vi "Read (Single Waveform).vi"(0 "VISA resource name":refnum<visa-resource-name>, 1 "Segment Index (0)":i32 format="%.0g", 5 "Measurement Source (1: Channel 1)":i32(ring)=1 items=["Channel 1"=1, "Channel 2"=2, "Channel 3"=3, "Channel 4"=4, "Function 1"=5, "Function 2"=6, "Function 3"=7, "Function 4"=8, "Memory 1"=9, "Memory 2"=10, "Memory 3"=11, "Memory 4"=12], 9 "Maximum Time (100000ms)":u32=100000, 11 "error in (no error)":errorcluster) -> (4 "VISA resource name out":refnum<visa-resource-name>, 8 "Waveform Data":waveform(dbl)(graph), 15 "error out":errorcluster)   [LabVIEW 2020, in "Agilent 90000 Series.lvlib"]
doc: "Initiates an acquisition on all channels that you enabled with the Configure Channel VI. The VI waits for the acquisition to complete and returns the waveform for the <B>Measurement Source</B> you specified. If the oscilloscope did not complete the acquisition within the time period you specify with the <B>Maximum Time</B> control, the VI returns a timeout error. A common cause for a timeout error is the acquisition was not triggered. For example, the trigger level is out of range of the waveform. If the sampling mode is set to segment, you can set the <B>Segment Index</B>.\n\nCall the Fetch (Single Waveform) VI to obtain the waveforms for each of the remaining enabled channels without initiating another acquisition.\n\n<B>Note:</B> If your instrument does not support auto compensation for probe attenuation, you may need to adjust the scaling of the Waveform Data accordingly. This is handled automatically in the <B>Configure Channel</B> VI or can be done manually by multiplying the <B>Waveform Data</B> by the probe attenuation."
uses:
  Agilent 90000 Series.lvlib
  Low Level/Fetch (Waveform).vi
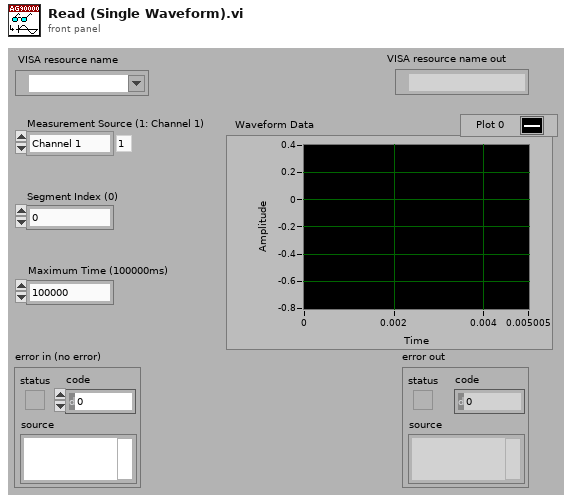
[diagram p1: front panel]
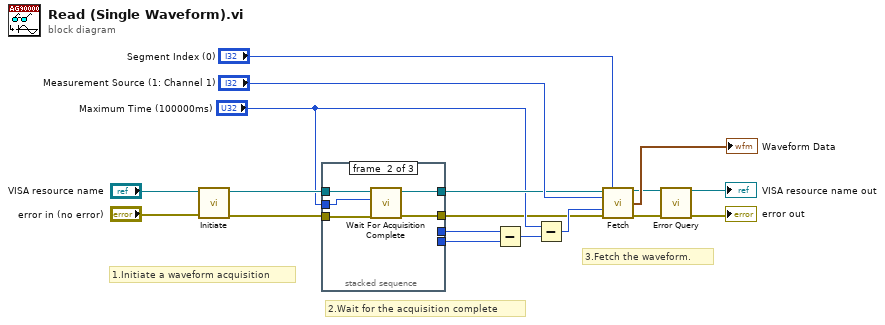
[diagram p0: block diagram]
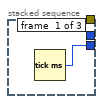
[diagram p2: hidden frame]
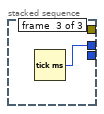
[diagram p3: hidden frame]
diagram:
  # "3.Fetch the waveform."
  # "2.Wait for the acquisition complete"
  # "1.Initiate a waveform acquisition"
  n1 = call "Initiate.vi"("error in (no error)"="error in (no error)", "VISA resource name"="VISA resource name") -> ("error out"=w8:errorcluster, "VISA resource name out"=w9:refnum<visa-resource-name>)  [unwired: 8 out]
  n2 = stacked-sequence {
    tunnel: [w19 _ _] -> w3
    tunnel: [_ _ w25] -> w4
    tunnel: w9 -> [_ w21 _]
    tunnel: [_ w24 _] -> w7
    tunnel: w8 -> [_ w22 _]
    tunnel: [_ w23 _] -> w1
    tunnel: "Maximum Time (100000ms)" -> [_ w20 _]
    frame #0 {
      n3 = Tick Count (ms)() -> (millisecond timer value=w19:u32)
    }
    frame #1 {
      n4 = call "Wait For Acquisition Complete.vi"("error in (no error)"=w22, "Maximum Time (10000ms)"=w20, "VISA resource name"=w21) -> ("error out"=w23:errorcluster, "VISA resource name out"=w24:refnum<visa-resource-name>)  [unwired: 7 out]
    }
    frame #2 {
      n5 = Tick Count (ms)() -> (millisecond timer value=w25:u32)
    }
  }
  n6 = Subtract(x=w4, y=w3) -> (x-y=w6:u32)
  n7 = Subtract(x="Maximum Time (100000ms)", y=w6) -> (x-y=w2:u32)
  n8 = call-poly "Fetch.vi"("VISA resource name"=w7, "Segment Index (0)"="Segment Index (0)", "Measurement Source (1: Channel 1)"="Measurement Source (1: Channel 1)", "Maximum Time (10000ms)"=w2, "error in (no error)"=w1) -> ("VISA resource name out"=w11:refnum<visa-resource-name>, "Waveform Data"=→"Waveform Data":waveform(dbl), "error out"=w10:errorcluster)  [unwired: 8 out]
  n9 = call "Error Query.vi"("error in (no error)"=w10, "VISA resource name"=w11) -> ("error out"=→"error out":errorcluster, "VISA resource name out"=→"VISA resource name out":refnum<visa-resource-name>)  [unwired: 8 out]
